vi "ChannelSettings.vi"(6 "Operation":T1, 7 "error in (no error)":errorcluster, 10 "Value_IN":string[][](array[string])) -> (0 "error out":errorcluster, 1 "Scale":dbl[](array[numeric]), 2 "Offset":dbl[](array[numeric]), 3 "Name":string[](array[string]), 4 "Value_OUT":string[][](array[string]))   [LabVIEW 2011]
uses:
  Strict Type Controls/Settings Operation.ctl
  <vilib>/Utility/file.llb/Read From Spreadsheet File (string).vi
  <vilib>/Utility/file.llb/Write To Spreadsheet File (string).vi
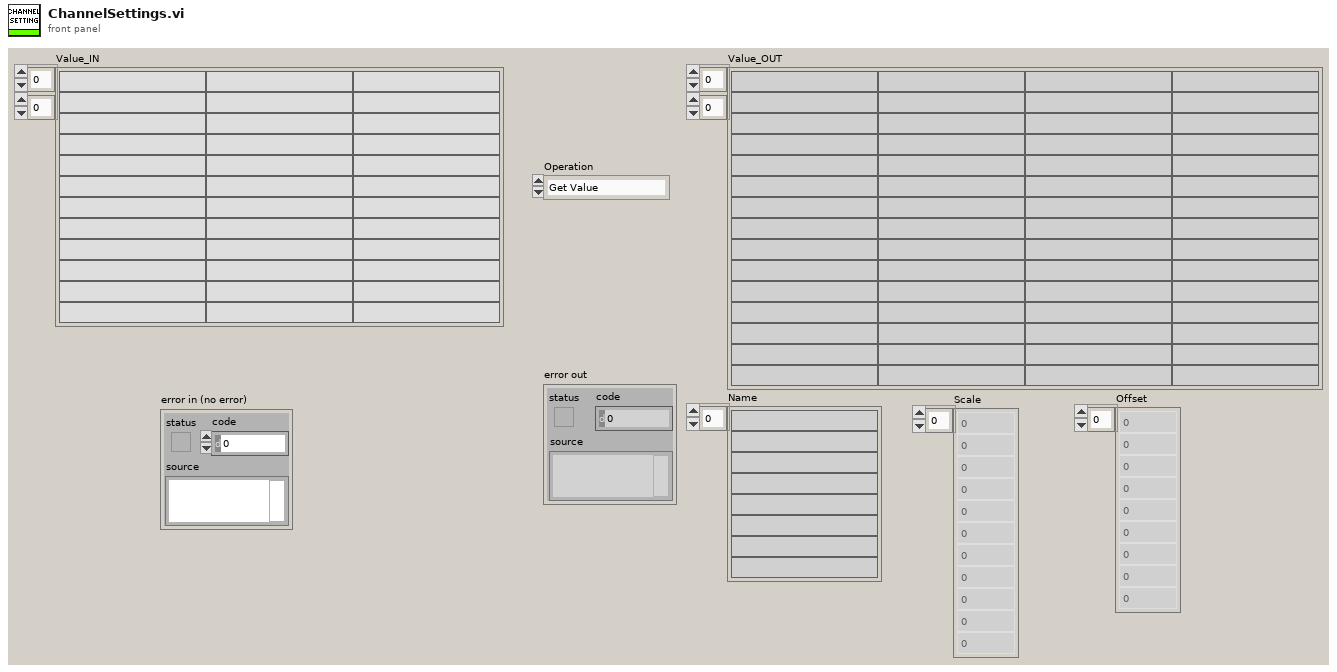
[diagram p1: front panel]
types:
  T1 = typedef "Settings Operation.ctl" = enum8{"Get Value", "Set Value", "Read File", "Write File", "Write Stored Value"}
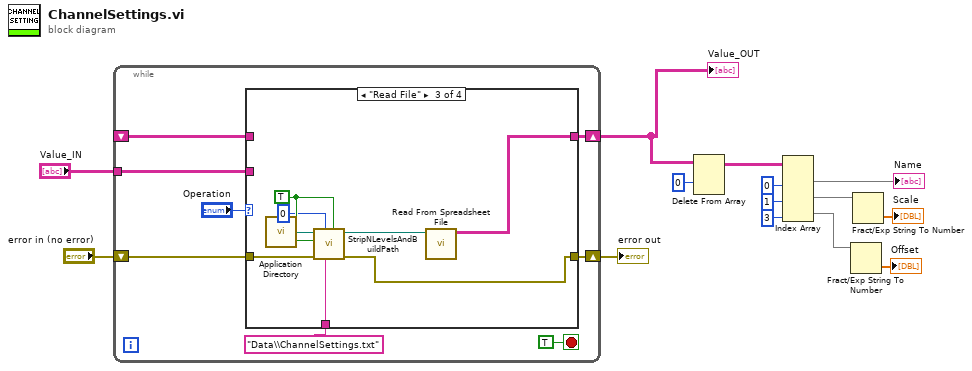
[diagram p0: block diagram]
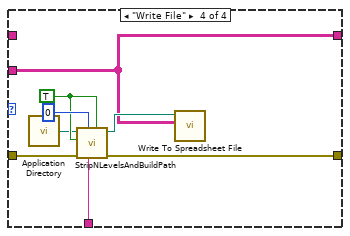
[diagram p4: hidden frame]
diagram:
  n1 = while {
    shift-right: [w21] -> w11
    shift-left: _ -> [w22]
    shift-right: [w19] -> w13
    shift-left: "error in (no error)" -> [w20]
    tunnel: "Value_IN" -> [w15]
    stop <- TRUE stop-if-true
    n2 = case shown="\"Read File\"" "Operation" {
      tunnel: w22 -> [w24 _ _ _]
      tunnel: [w24 w25 w27 w36] -> w21
      tunnel: w20 -> [w23 w26 w34 w42]
      tunnel: [w23 w26 w28 w35] -> w19
      tunnel: "Data\\ChannelSettings.txt" ("Build Path") -> [_ _ w33 w41]
      tunnel: w15 -> [_ w25 _ w36]
      frame "Get Value", Default {
      }
      frame "Set Value" {
      }
      frame "Read File" {
        w31 = TRUE ("Is File?")
        n3 = call <vilib>:"Application Directory.vi"() -> ("Application Directory"=w32:path)
        n4 = call "StripNLevelsAndBuildPath.vi"("Create Folders"=w31, "Build Path"=w33, "Strip Levels"=0, "error in(no error)"=w34, "Is File"=w31, "Path In"=w32) -> ("error out"=w28:errorcluster, "Path Out"=w29:path)  [unwired: 4 in]
        n5 = call-poly <vilib>:"Read From Spreadsheet File.vi"("file path (dialog if empty)"=w29) -> ("all rows"=w27:string[][])  [unwired: 6 in, 4 out]
      }
      frame "Write File" {
        w39 = TRUE ("Is File?")
        n6 = call <vilib>:"Application Directory.vi"() -> ("Application Directory"=w38:path)
        n7 = call "StripNLevelsAndBuildPath.vi"("Create Folders"=w39, "Build Path"=w41, "Strip Levels"=0, "error in(no error)"=w42, "Is File"=w39, "Path In"=w38) -> ("error out"=w35:errorcluster, "Path Out"=w37:path)  [unwired: 4 out]
        n8 = call-poly <vilib>:"Write To Spreadsheet File.vi"("2D data"=w36, "file path (dialog if empty)"=w37) -> ()  [unwired: 6 in, 1 out]
      }
    }
  }
  "error out" <- w13
  "Value_OUT" <- w11
  n9 = Delete From Array(array=w11, index (row)=0) -> (array with subset deleted=w10:string[][])  [unwired: 2 in, 1 out]
  n10 = Index Array(array=w10, index (col) #1=0 ("disabled index (col)"), index (col) #2=1 ("index (col)"), index (col) #3=3 ("index (col)")) -> (element #1=→"Name":string[], element #2=w4:string[], element #3=w3:string[])  [unwired: 3 in]
  n11 = Fract/Exp String To Number(string=w3) -> (number=→"Offset":dbl[])  [unwired: 3 in, 1 out]
  n12 = Fract/Exp String To Number(string=w4) -> (number=→"Scale":dbl[])  [unwired: 3 in, 1 out]
